vi "Global.vi"() -> ()   [LabVIEW 2020]
panel:
  out "机台号":string
  out "参数1":string[](array[string])
  out "保存条件1":bool
  out "Path":string
  out "实时压力":string
  out "start_time":string
  out "test_station_name":string
  out "station_id":string
  out "test_station":string
  out "产品进站":bool
  out "RecordDate":string
  out "接口调用频率":u32
  out "正在运行":bool
  out "待机超限时间":u32
  out "强制停止":bool
  out "MES状态":bool
  in  "MES参数":T1
  in  "运行状态位置":i32
  out "audit_mode":string
  out "product":string
  out "model":string
  out "运行状态时间点":dbl[](array[numeric])
  out "sn":string
  out "tsid":string
  out "mes抬头":string[][](array[string])
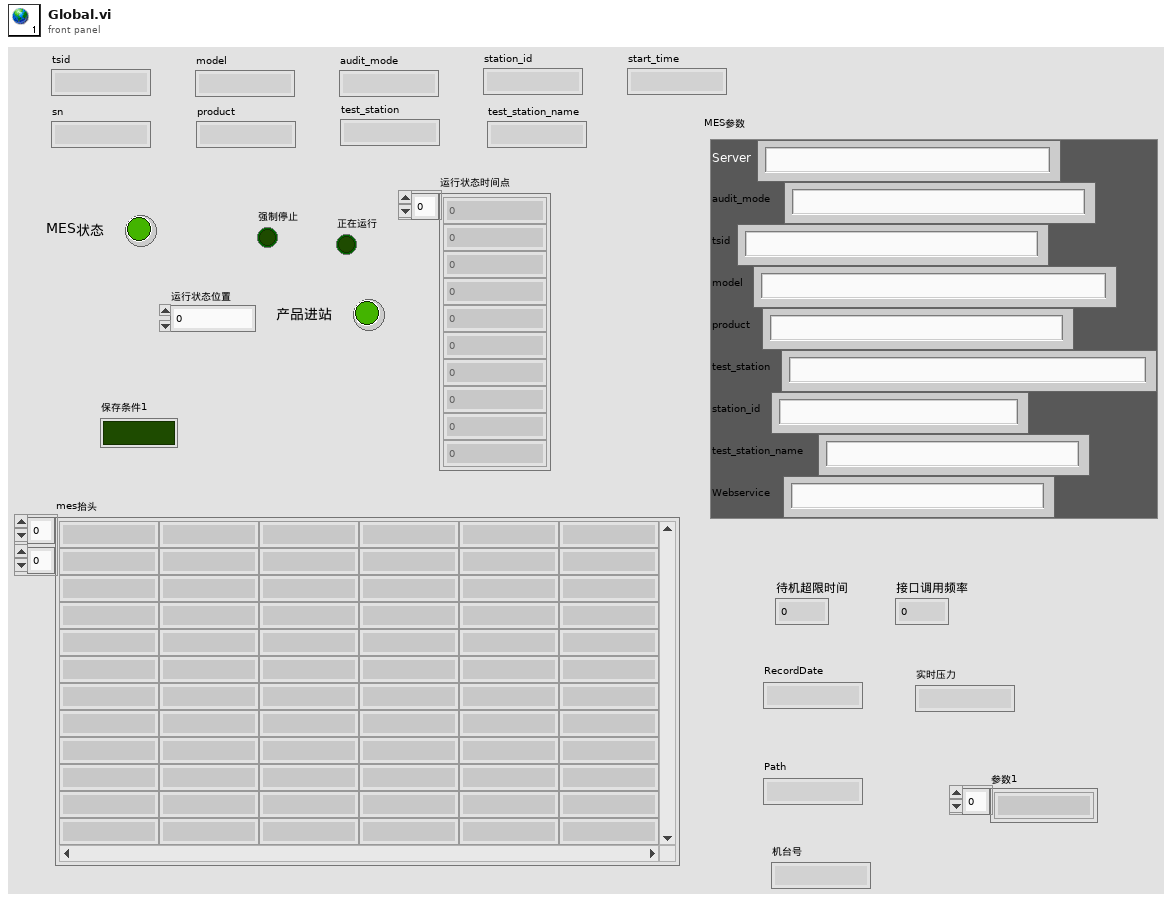
[diagram p1: front panel]
types:
  T1 = cluster{"Server":string, "audit_mode":string, "tsid":string, "model":string, "product":string, "test_station":string, "station_id":string, "test_station_name":string, "Webservice":string}
diagram:
